vi "Relabel.vi"(10 "Relabel messages with":string) -> (3 "Translator":refnum<class "Relabel.lvclass">)   [LabVIEW 2011, in "Messenging.lvlib" / "Relabel.lvclass"]
uses:
  Relabel.lvclass
  Relabel.lvclass/Relabel.ctl
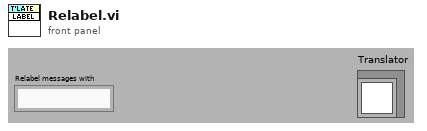
[diagram p1: front panel]
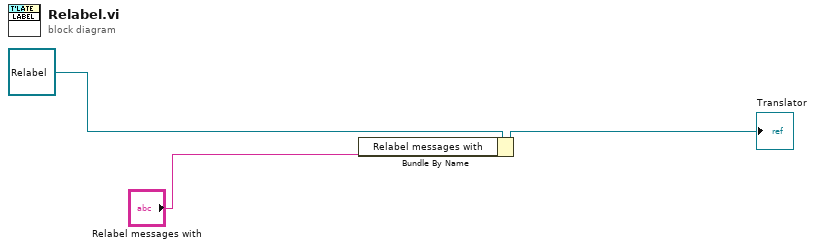
[diagram p0: block diagram]
diagram:
  n1 = Bundle By Name(cluster=refnum<class "Relabel.lvclass"> refnum ("SubstututeMessage in"), "Relabel messages with"="Relabel messages with") -> (→"Translator":refnum<class "Relabel.lvclass">)
